vi "make lockin params.vi"(7 "self":enum16{"Diode", "RF mixer", "lockin"}(ring), 9 "scope settings":T1, 11 "Lockin":cluster{"LP BW (kHz)":dbl, "notch BW (kHz)":dbl}={"LP BW (kHz)"=5.0, "notch BW (kHz)"=2.0}) -> (3 "param Lockin":T2)   [LabVIEW 2018]
uses:
  scope settings.ctl
  <vilib>/rvi/Analysis/host/Butterworth/config/Butterworth Filter Order.ctl
  <vilib>/rvi/Analysis/host/Butterworth/config/Butterworth Filter Type.ctl
  <vilib>/rvi/Analysis/host/Butterworth/config/BwScaledCoefficients.vi
  <vilib>/rvi/Analysis/host/Notch/config/NotchScaledCoefficients.vi
  <vilib>/rvi/Analysis/host/Butterworth/XNode/ButterworthCoefficients.xnode
  <vilib>/rvi/Analysis/host/Notch/XNode/NotchCoefficients.xnode
  <vilib>/rvi/Analysis/host/Public/NI_FpgaMspHost.lvlib
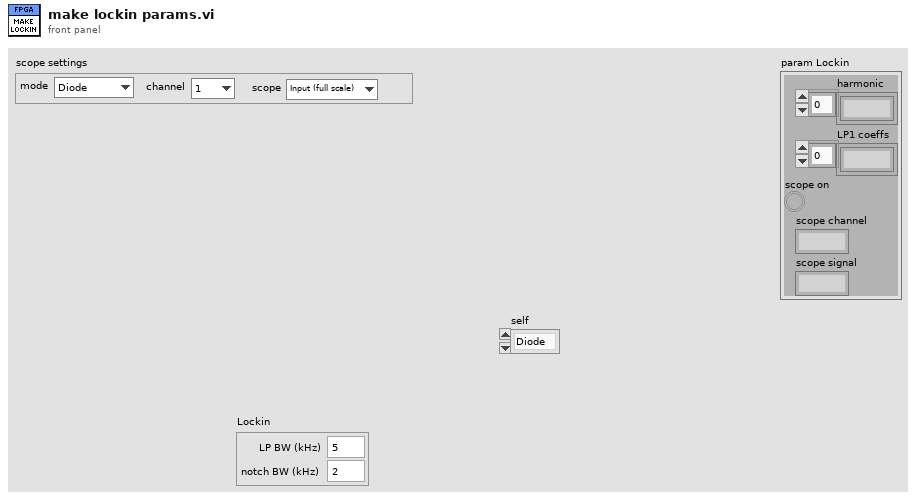
[diagram p1: front panel]
types:
  T1 = typedef "scope settings.ctl" = cluster{"mode":enum16{"Diode", "RF mixer", "lockin"}, "channel":enum16{"1", "2", "3"}, "scope":enum16{"Input (full scale)", "PLL out", "Phase error (deg)", "Freq. error (Hz)"}}
  T2 = cluster{"harmonic":fxp<+,20,6>[], "LP1 coeffs":i32[], "scope on":bool, "scope channel":u8, "scope signal":u8}
  T3 = enum16{"Input (full scale)", "PLL out", "Phase error (deg)", "Freq. error (Hz)"}
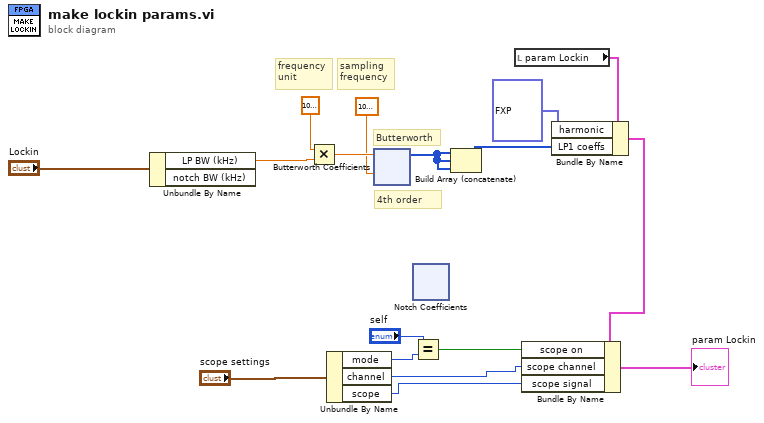
[diagram p0: block diagram]
diagram:
  # "4th order"
  # "Butterworth"
  # "frequency\nunit"
  # "sampling\nfrequency"
  n1 = Unbundle By Name("Lockin") -> ("LP BW (kHz)"=w14:dbl)  [unwired: 1 out]
  n2 = Multiply(x=1000.0 ("sample rate (S/s)"), y=w14) -> (x*y=w17:dbl)
  n3 = Unbundle By Name("scope settings") -> ("mode"=w8:enum16{"Diode", "RF mixer", "lockin"}, "channel"=w5:enum16{"1", "2", "3"}, "scope"=w4:T3)
  n4 = xnode "Butterworth Coefficients"("cutoff frequency (Hz)"=w17, "sample rate (S/s)"=1000000.0) -> ("scaled coefficients"=w13:i32[])  [unwired: 1 in, 1 out]
  n5 = xnode "Notch Coefficients"() -> ()  [unwired: 4 in, 2 out]
  n6 = Equal?(x="self", y=w8) -> (x = y?=w6:bool)
  n7 = Build Array (concatenate)(w13, w13, w13) -> (w11:i32[])
  n8 = local read "param Lockin"() -> (w12:T2)
  n9 = Bundle By Name(cluster=w12, "harmonic"=fxp<+,20,6>[] [2.0, 2.0, 2.0], "LP1 coeffs"=w11) -> (w2:T2)
  n10 = Bundle By Name(cluster=w2, "scope on"=w6, "scope channel"=w5, "scope signal"=w4) -> (→"param Lockin":T2)
